vi "Get Row Values.vi"(7 "Sheet Name":string, 8 "error in":errorcluster, 10 "Row Address":string="A1", 11 "SpreadsheetDoc in":refnum<k24>) -> (0 "error out":errorcluster, 1 "Types":T1[](array[typedef]), 2 "Cell Values":T2(array[cluster]) {"Time Stamp" format="%<%x %.3X>T"}, 3 "SpreadsheetDoc out":refnum<k24>)   [LabVIEW 2019, in "Open Xml.lvlib"]
doc: "Returns all defined cells in a row"
uses:
  Open Xml.lvlib
  D:/git/Open-Xml-LabVIEW/Source/DocumentFormat.OpenXml.dll
  DocumentFormat.OpenXml.dll
  Cell DataType.ctl
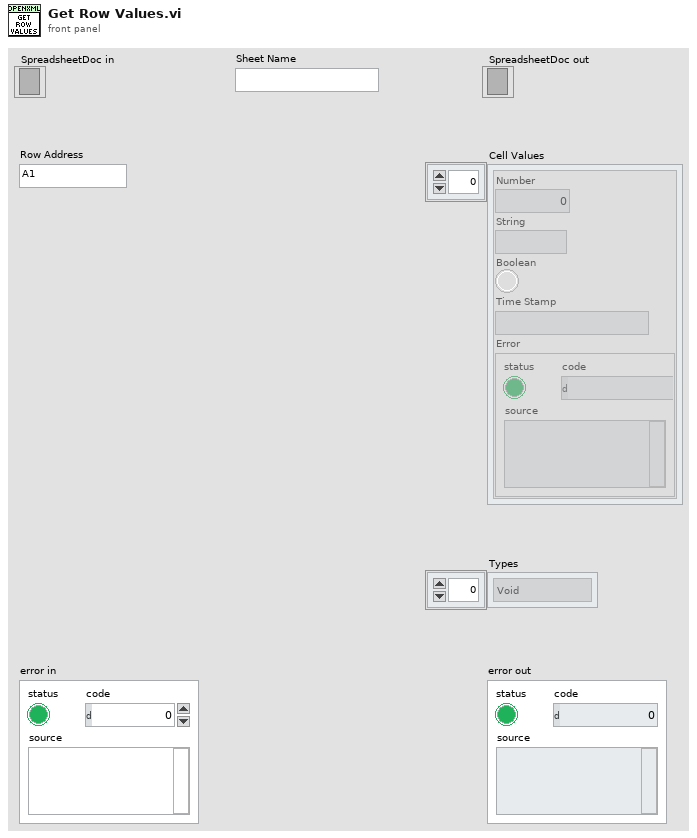
[diagram p1: front panel]
types:
  T1 = typedef "Open Xml.lvlib/Cell DataType.ctl" = enum16{"Void", "Boolean", "Number", "Error", "SharedString", "String", "InlineString", "Date"}
  T2 = cluster{"Number":dbl, "String":string, "Boolean":bool, "Time Stamp":timestamp, "Error":errorcluster}[]
  T3 = cluster{"Number":dbl, "String":string, "Boolean":bool, "Timestamp":timestamp, "Error":errorcluster}
  T4 = cluster{"Number":dbl, "String":string, "Boolean":bool, "Timestamp":timestamp, "Error":errorcluster}[]
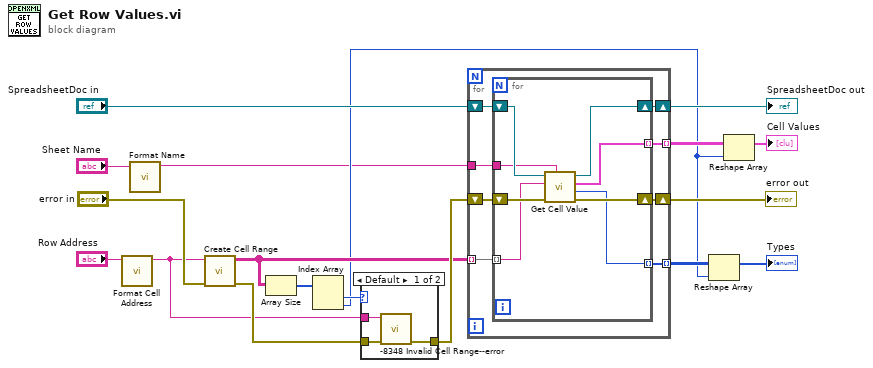
[diagram p0: block diagram]
diagram:
  n1 = call "Format Cell Address.vi"("Cell Address"="Row Address") -> ("Formatted Cell Address"=w4:string)  [unwired: 10 in]
  n2 = call "Format Name.vi"("Sheet Name"="Sheet Name") -> ("Formatted Sheet Name"=w1:string)  [unwired: 10 in]
  n3 = call "Create Cell Range.vi"("error in"="error in", "Cell Range"=w4) -> ("error out"=w14:errorcluster, "Cell Range"=w11:string[][])  [unwired: 8 in]
  n4 = Array Size(array=w11) -> (size(s)=w10:i32[])
  n5 = Index Array(array=w10) -> (element #1=w9:i32, element #2=w5:i32)  [unwired: 2 in]
  n6 = case shown="Default" w9 {
    tunnel: w14 -> [w21 w22]
    tunnel: [w20 w22] -> w12
    tunnel: w4 -> [w19 _]
    frame Default {
      n7 = call "-8348 Invalid Cell Range--error.vi"("error in"=w21, "Argument"=w19) -> ("error out"=w20:errorcluster)  [unwired: 9 in]
    }
    frame 1 {
    }
  }
  n8 = for {
    tunnel: w11 -> [w28] mode=indexing
    tunnel: [w26] -> w7 mode=indexing
    tunnel: [w25] -> w15 mode=indexing
    shift-right: [w29] -> w17
    shift-left: "SpreadsheetDoc in" -> [w27]
    shift-right: [w30] -> w18
    shift-left: w12 -> [w24]
    tunnel: w1 -> [w23]
    n9 = for {
      tunnel: [w34] -> w26 mode=indexing
      tunnel: [w31] -> w25 mode=indexing
      shift-right: [w35] -> w30
      shift-left: w24 -> [w36]
      shift-right: [w37] -> w29
      shift-left: w27 -> [w38]
      tunnel: w28 -> [w32] mode=indexing
      tunnel: w23 -> [w33]
      n10 = call "Get Cell Value.vi"("Sheet Name"=w33, "error in"=w36, "Cell Address"=w32, "SpreadsheetDoc in"=w38) -> ("error out"=w35:errorcluster, "Type"=w31:T1, "Cell Value"=w34:T3, "SpreadsheetDoc out"=w37:refnum<k24>)  [unwired: 4 in]
    }
  }
  "SpreadsheetDoc out" <- w17
  "error out" <- w18
  n11 = Reshape Array(w15, w5) -> (→"Types":T1[])
  n12 = Reshape Array(w7, w5) -> (→"Cell Values":T4)
